vi "三菱全局变量.vi"() -> ()   [LabVIEW 2014]
panel:
  in  "串口设置":T1={"通讯串口"="COM1", "波特率"=9600, "数据比特"=8, "奇偶校验"=enum."None", "停止位"=10, "等待延时(ms)"=0} {"停止位" items=["1.0"=10, "1.5"=15, "2.0"=20]; "数据比特" min=5 max=8 step=1; "波特率" items=["75"=75, "110"=110, "134"=134, "150"=150, "300"=300, "600"=600, "1200"=1200, "1800"=1800, "2400"=2400, "4800"=4800, "7200"=7200, "9600"=9600, "14400"=14400, "19200"=19200, "28800"=28800, "38400"=38400, "56000"=56000, "57600"=57600, "115200"=115200, "128000"=128000, "230400"=230400]}
  out "关闭串口":bool
  out "PC->PLC D寄存器":i16[](array[numeric])
  out "PLC->PC D寄存器":i16[](array[numeric])
  in  "写Y寄存器长度":u16
  in  "写寄存器开始地址":u16
  in  "读X寄存器长度":u16
  in  "读X寄存器开始地址":u16
  in  "读D寄存器长度":u16
  in  "读D寄存器开始地址":u16
  in  "写D寄存器长度":u16
  in  "写D寄存器开始地址":u16
  out "通讯失败":bool
  out "打开串口":bool
  out "退出":bool
  in  "通讯":T2(ring)
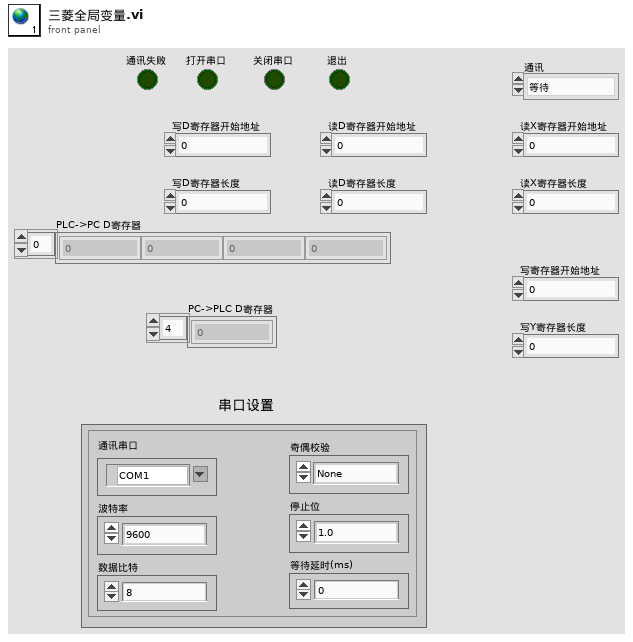
[diagram p1: front panel]
types:
  T1 = cluster{"通讯串口":refnum<visa-resource-name>, "波特率":u32, "数据比特":u16, "奇偶校验":enum16{"None", "Odd", "Even", "Mark", "Space"}, "停止位":u16, "等待延时(ms)":u32}
  T2 = enum16{"等待", "打开串口", "关闭串口", "通讯失败", "读数据", "写数据"}
diagram:
